vi "Measurement UI.vi"() -> ()   [LabVIEW 2024, in "OneShot-PureTone UI.lvlib"]
uses:
  OneShot-PureTone UI.lvlib
  <vilib>/addons/_XControls/Spectrum with Cursors/Spectrum with Cursors.xctl
  <vilib>/addons/_NISVFA/_Shared subVIs/Data Objects/Data/Data.lvclass
  <vilib>/Addons/_XControls/Waveforms with Cursors/Waveforms with Cursors.xctl
  <vilib>/addons/_NISVFA/_Shared subVIs/Controls/svc_Window.ctl
  <vilib>/addons/_NISVFA/_Shared subVIs/Data Objects/Data/Data.lvclass/Data.ctl
  <vilib>/addons/_NISVFA/_Shared subVIs/Common/SVL Set dB Reference (1 Ch).vi
  <vilib>/addons/Sound and Vibration/svt_Level/SVL AC & DC Level (Time) (1 Ch).vi
  <vilib>/addons/Sound and Vibration/svt_Single Tone Measurements/SVT Spurious Free Dynamic Range (Frequency) (1 Ch).vi
  <vilib>/addons/_NISVFA/_Shared subVIs/Data Objects/Y (Complex) (DBL)/SV Convert Complex Spectrum to Data Object.vi
  <vilib>/addons/_NISVFA/_Shared subVIs/Common/SVL Set dB Reference (variant).vi
  <vilib>/addons/_NISVFA/_Shared subVIs/Common/svc_Get SV Channel Info.vi
  <vilib>/Analysis/baseanly.llb/Mean.vi
  <vilib>/Analysis/baseanly.llb/Mean (DBL).vi
  <vilib>/addons/_NISVFA/_Shared subVIs/Windowing/svfa_Scaled Time Domain Window (Array).vi
  <vilib>/addons/_NISVFA/_Spectrum Processing/SVFA Get Spectrum Subset.vi
  <vilib>/addons/_NISVFA/_Spectrum Processing/SVFA Get Spectrum Subset (Complex) (1 Ch).vi
  <vilib>/addons/_NISVFA/_Shared subVIs/Common/svc_Window Parameters.vi
  <vilib>/addons/_NISVFA/_Shared subVIs/Common/svc_Extract Single Tone Information (complex).vi
  <vilib>/addons/_NISVFA/_Shared subVIs/Common/svc_Check Frequency Range in Spectrum.vi
  <vilib>/addons/_NISVFA/_Spectrum Processing/SVFA Unit Conversion.vi
  <vilib>/addons/_NISVFA/_Spectrum Processing/SVFA Unit Conversion (Complex) (1 Ch).vi
  <vilib>/addons/_NISVFA/_Spectrum Processing/SVFA Spectrum Peak Search.vi
  <vilib>/addons/_NISVFA/_Spectrum Processing/SVFA Spectrum Peak Search (1 Ch).vi
  <vilib>/addons/_NISVFA/_Shared subVIs/Common/svc_Spectrum Units.vi
  <vilib>/addons/_NISVFA/_Shared subVIs/Common/sv_Get NI Property Name String.vi
  <vilib>/addons/_NISVFA/_Shared subVIs/Data Objects/Data/Write Data Attributes.vi
  <vilib>/addons/_NISVFA/_Shared subVIs/Common/svc_Unit Label to Engineering Units.vi
  <vilib>/addons/_NISVFA/_Shared subVIs/Common/svc_Engineering Units to Unit Label.vi
  <vilib>/addons/_NISVFA/_Spectrum Processing/subVIs/svfa_Spectrum Info Window to windowTd Type Def.vi
  <vilib>/Analysis/4window.llb/Force Window.vi
  <vilib>/Analysis/4window.llb/Force Window (DBL).vi
  <vilib>/Analysis/4window.llb/Exponential Window.vi
  <vilib>/Analysis/4window.llb/Exponential Window (DBL).vi
  <vilib>/addons/_NISVFA/_Shared subVIs/Common/svc_Build Unit Label for Frequency Range.vi
  <vilib>/addons/_NISVFA/_Spectrum Processing/SVFA Get Tone Amplitude and Phase (1 Ch).vi
  <vilib>/addons/_NISVFA/_Spectrum Processing/subVIs/svfa_Compute Complex Spectrum for Export.vi
  <vilib>/addons/_NISVFA/_Shared subVIs/Common/svc_Check Frequency Range in Bandwidth.vi
  <vilib>/addons/_NISVFA/_Shared subVIs/Common/svc_Convert Start and Stop to Start Index and Length.vi
  <vilib>/addons/_NISVFA/_Shared subVIs/Common/svc_Log View for Spectrum (1Ch).vi
  <vilib>/addons/_NISVFA/_Spectrum Processing/SVFA Unit Conversion (1 Ch).vi
  <vilib>/addons/_NISVFA/_Shared subVIs/Common/svc_Complex Datatype Defaults.vi
  <vilib>/addons/_NISVFA/_Spectrum Processing/subVIs/svfa_Spectrum Peak Search.vi
  <vilib>/addons/_NISVFA/_Shared subVIs/Common/svc_Format Value (DBL).vi
  <vilib>/addons/_NISVFA/_Shared subVIs/Common/svc_Get Weighting Enum and Labels.vi
  <vilib>/addons/_NISVFA/_Shared subVIs/Common/svc_Surround NonAlpha String with Parentheses.vi
  <vilib>/dlg_ctls.llb/Space Constant.vi
  <vilib>/addons/_NISVFA/_Shared subVIs/Data Objects/Data/Read Data Attributes.vi
  <vilib>/addons/_NISVFA/_Spectrum Processing/subVIs/svfa_Window Frequency Response.vi
  <vilib>/addons/_NISVFA/_Spectrum Processing/subVIs/svfa_Window Frequency Response (double array).vi
  <vilib>/Analysis/baseanly.llb/Dot Product.vi
  <vilib>/Analysis/baseanly.llb/Complex Dot Product.vi
  <vilib>/addons/_NISVFA/_Shared subVIs/Common/svc_Unwrap Phase.vi
  <vilib>/addons/_NISVFA/_Shared subVIs/Common/svc_Convert Spectrum Array to dB.vi
  <vilib>/addons/_NISVFA/_Spectrum Processing/subVIs/svfa_Conversion Utility (spectrum info).vi
  <vilib>/addons/_NISVFA/_Spectrum Processing/subVIs/svfa_Peak Rough Search Indices.vi
  <vilib>/addons/_NISVFA/_Shared subVIs/Common/svc_Unit Label Lexical Class.vi
  <vilib>/addons/_NISVFA/_Spectrum Processing/subVIs/svfa_Rect Window Frequency Response.vi
  <vilib>/addons/_NISVFA/_Spectrum Processing/subVIs/svfa_Cosine Window Coefficients.vi
  <vilib>/addons/_NISVFA/_Spectrum Processing/subVIs/svfa_Peak to RMS to Peak2Peak.vi
  <vilib>/addons/_NISVFA/_Spectrum Processing/subVIs/svfa_Mag to Mag2.vi
  <vilib>/addons/_NISVFA/_Spectrum Processing/subVIs/svfa_Linear to dB.vi
  <vilib>/addons/_NISVFA/_Spectrum Processing/subVIs/svfa_dBrefA to dBrefB.vi
  <vilib>/addons/_NISVFA/_Spectrum Processing/subVIs/svfa_Spectrum to Spectral Density.vi
  <vilib>/addons/_NISVFA/_Shared subVIs/Data Objects/Y (Complex) (DBL)/Y (Complex) (1 Ch).lvclass
  <vilib>/addons/_NISVFA/_Shared subVIs/Common/svc_Caller VI Returned in Error Source.vi
  <vilib>/addons/_NISVFA/_Shared subVIs/Common/svc_Get Window Info.vi
  <vilib>/Analysis/0measdsp.llb/Scaled Time Domain Window.vi
  <vilib>/Analysis/0measdsp.llb/Scaled Time Domain Window (DBL).vi
  <vilib>/Utility/error.llb/Error Cluster From Error Code.vi
  <vilib>/Analysis/baseanly.llb/Std Deviation and Variance.vi
  <vilib>/addons/Sound and Vibration/svt_Single Tone Measurements/SVT Gain (Time) (1 Ch).vi
  <vilib>/addons/Sound and Vibration/svt_Distortion/SVT THD and Harmonic Components (Frequency) (1 Ch).vi
  <vilib>/addons/Sound and Vibration/svt_Distortion/SVT SNR without Harmonics (Frequency) (1 Ch).vi
  <vilib>/addons/Sound and Vibration/svt_Single Tone Measurements/SVT Dynamic Range (Frequency) (1 Ch).vi
  <vilib>/addons/Sound and Vibration/svt_Distortion/subVIs/sv_Check Data Valid (Audio) (1 Ch).vi
  <vilib>/addons/_NISVFA/_Shared subVIs/Common/svc_Convert Frequency to Frequency String.vi
  <vilib>/Analysis/4window.llb/window parameters.vi
  <vilib>/Analysis/4window.llb/Window Properties.vi
  <vilib>/Analysis/4window.llb/Window Properties by Name.vi
  <vilib>/addons/_NISVFA/_Spectrum Processing/subVIs/svfa_Spectrum Peak Tone Search and Estimation (complex).vi
  <vilib>/measure/masignal.llb/Tones and Noise Waveform.vi
  <vilib>/addons/_NISVFA/_Shared subVIs/Common/svc_FFT with Window.vi
  <vilib>/Analysis/1siggen.llb/Square Wave.vi
  <vilib>/addons/_NISVFA/_Spectrum Processing/subVIs/svfa_Three Finger Peak Search.vi
  <vilib>/addons/Sound and Vibration/svt_Distortion/subVIs/sv_Peak View Amplitude (1 Ch).vi
  <vilib>/addons/_NISVFA/_Shared subVIs/Data Objects/Y (Complex) (DBL)/Write Y.vi
  <vilib>/addons/_NISVFA/_Shared subVIs/Spectrum Info/sv_Convert Spectrum Info to Variant Attributes.vi
  <vilib>/addons/Sound and Vibration/svt_Distortion/SoundVib_Distortion.lvlib
  <vilib>/addons/Sound and Vibration/svt_Single Tone Measurements/SoundVib_SingleTone.lvlib
panel:
  out "Waveforms with Cursors":waveform(dbl)[](xcontrol)
  out "THD maximum harmonic out":i32=9 min=-1 max=1000
  out "measurement subset dt":dbl
  out "measurement subset t0":dbl
  out "acquired response dt":dbl
  out "acquired response t0":dbl
  out "measurement subset":dbl[](array[numeric])
  out "acquired response":dbl[](array[numeric])
  out "band stop (Hz) out":dbl=20000.0 format="%.2f"
  out "band start (Hz) out":dbl=20.0 format="%.2f"
  out "detected frequency (Hz)":dbl=1000.0 min=20.0 max=100000.0 step=1.0 format="%.2f"
  out "Spectrum with Cursors":refnum<class "Data.lvclass">(xcontrol)
  out "detected amplitude":dbl=1.0 format="%.3g"
  in  "Tab Control":T1(tab)
  in  "output channel":string="Dev1/ao0"
  in  "ao pure tone channel (I/O)":tag caption="output channel"
  in  "AI range":dbl=-3.0 caption="ai range" format="±  %.3g V"
  in  "ai response channel (I/O)":tag caption="input channel"
  in  "input channel":string="Dev1/ai0"
  in  "sample rate (Hz)":dbl=51200.0 caption="sample rate" min=0.0 format="%#.2p Hz"
  in  "settle cycles":dbl=2.0 min=0.0 format="%#_g cycles"
  in  "settle time (s)":dbl=0.01 caption="settling" format="%#_3g s"
  in  "measurement cycles":dbl=20.0 min=1.0 format="%#_g cycles"
  in  "measurement duration (s)":dbl=0.1 caption="measurement" format="%#_3g s"
  in  "frequency (Hz)":dbl=997.0 caption="frequency" format="%_4f Hz"
  in  "amplitude":dbl=1.0 format="%_4g V"
  in  "THD maximum harmonic":i32=9 caption="THD max harmonic" min=-1 max=1000
  in  "band start (Hz)":dbl=20.0 caption="band start" format="%#_3p Hz"
  in  "band stop (Hz)":dbl=20000.0 caption="band stop" format="%#_3p Hz"
  in  "full scale (V pk)":dbl=2.0 caption="full scale" format="%#_3g V"
  out "SFDR (dB)":dbl caption="SFDR" format="%.1f dB"
  out "Dynamic Range (dB FS)":dbl caption="dynamic range" format="%.1f dB FS"
  out "THD+N (dB)":dbl caption="THD+N" format="%.1f dB"
  out "THD (%)":dbl caption="THD" format="%_4f %"
  out "SNR (dB)":dbl caption="SNR" format="%.1f dB"
  out "fundamental frequency (Hz)":dbl caption="fundamental frequency" format="%_6g Hz"
  out "fundamental amplitude (V)":dbl caption="fundamental amplitude" format="%_6g V"
  out "gain (dB)":dbl caption="gain" format="%.3f dB"
  out "THD (dB)":dbl caption="THD" format="%.1f dB"
  out "processing error":errorcluster
  # "These settings can be changed to remeasure \ndistortion and noise on existing response data."
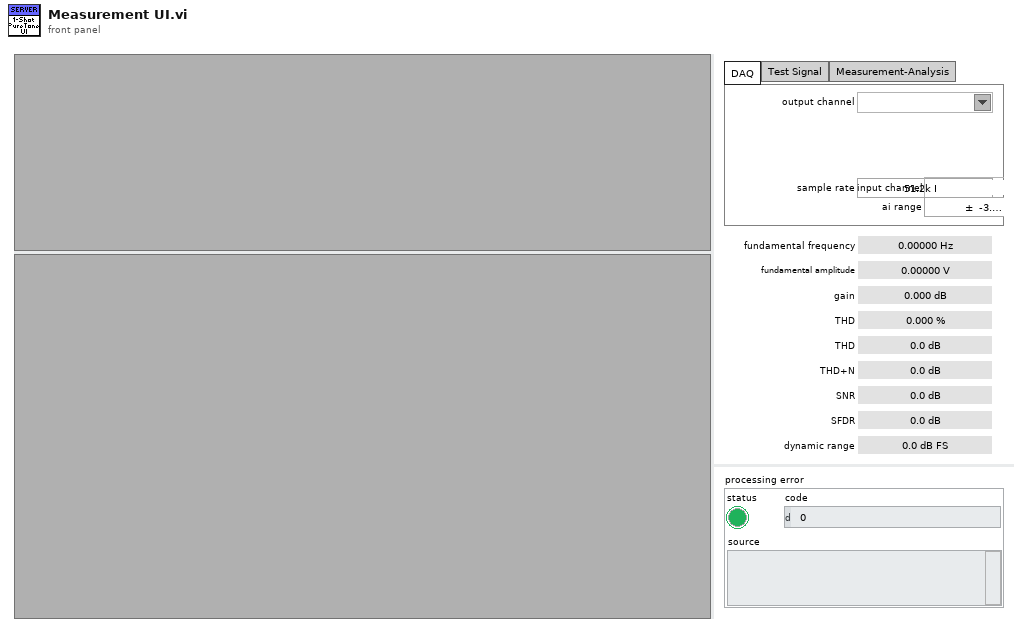
[diagram p1: front panel]
types:
  T1 = enum32{"DAQ", "Test Signal", "Measurement-Analysis"}
  T2 = cluster{"SNR units":enum16{"dB", "linear ratio", "%"}, "detected fundamental amplitude units":enum16{"EU rms", "EU peak", "EU peak-peak"}}
  T3 = cluster{"THD units":enum16{"dB", "linear ratio", "%"}, "harmonic component amplitude units":enum16{"EU rms", "EU peak", "EU peak-peak", "dB ref fund"}, "detected fundamental amplitude units":enum16{"EU rms", "EU peak", "EU peak-peak"}}
  T4 = cluster{"gain units":enum16{"dB", "linear ratio"}, "detected fundamental amplitude units":enum16{"EU rms", "EU peak", "EU peak-peak"}}
  T5 = typedef "svc_Window.ctl" = u32
  T6 = cluster{"band start (Hz)":dbl, "band stop (Hz)":dbl}
  T7 = typedef "svc_Spectrum Info.ctl" = cluster{"channel name":string, "description":string, "x-axis units":T8, "spectral info":cluster{"spectrum type":T9, "linear/dB":enum16{"linear", "dB"}, "window":u16, "window size":i32, "FFT size":i32}, "engineering units":T10, "custom label":string, "dB reference [EU]":dbl, "peak units":enum16{"rms", "peak", "peak-peak"}, "weighting filter":T11, "spectral density?":bool, "unit label":string, "spectrum skewed?":bool, "complimentary spectrum units":T12}
  T8 = typedef "svc_X-Axis Units.ctl" = u16
  T9 = typedef "svc_Spectrum Type.ctl" = enum16{"FFT Spectrum [complex]", "Amplitude [Magnitude]", "Power [Magnitude^2]", "Cross Spectrum [complex]", "Frequency Response [Complex]"}
  T10 = typedef "svc_Engineering Units Text Ring.ctl" = u16
  T11 = typedef "svc_Weighting Filter Text Ring.ctl" = u16
  T12 = typedef "svc_Complimentary Spectrum Units.ctl" = enum16{"none", "radians", "degrees", "cycles", "imaginary"}
  T13 = cluster{"complex spectrum response":cluster{"f0":dbl, "df":dbl, "complex spectrum":cdb[]}, "spectrum info":T7}
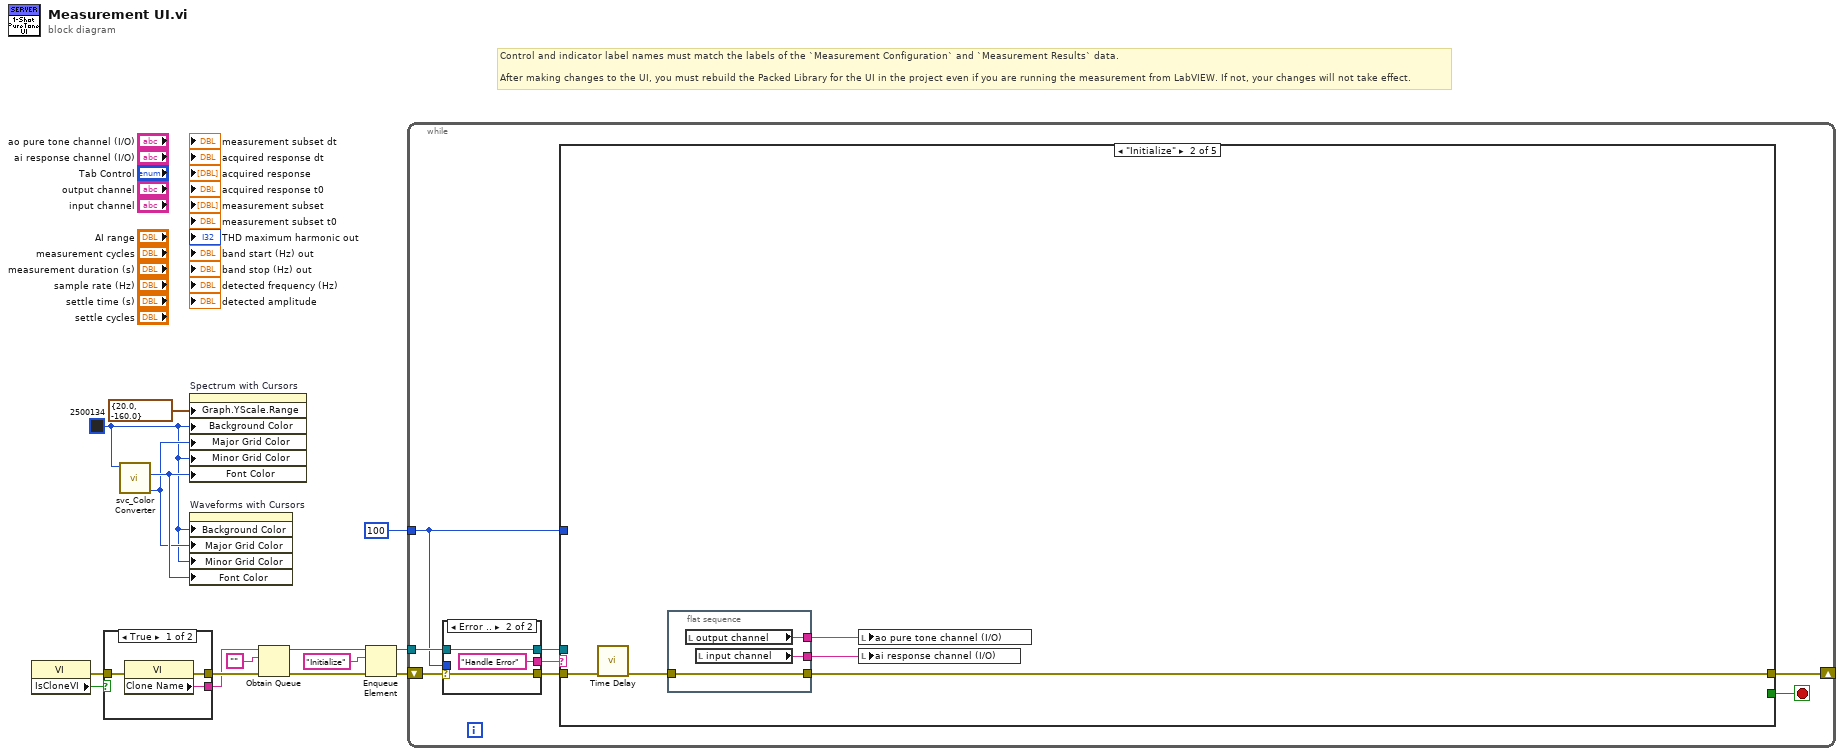
[diagram p0: block diagram]
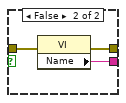
[diagram p2: hidden frame]
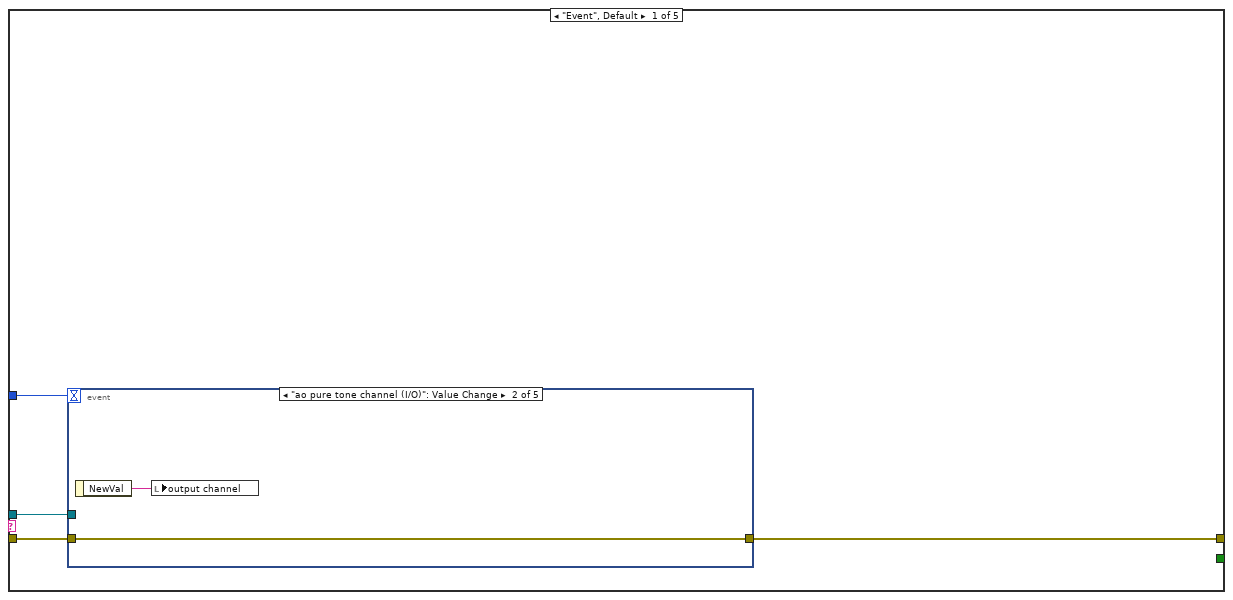
[diagram p3: hidden frame]
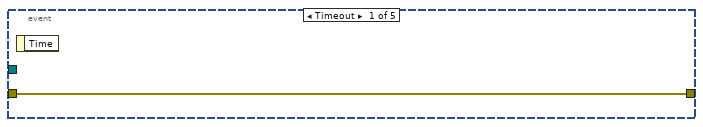
[diagram p4: hidden frame]
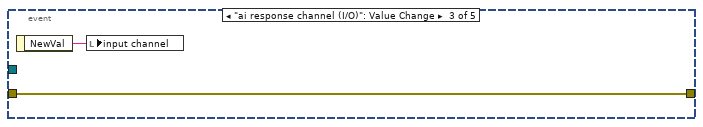
[diagram p5: hidden frame]
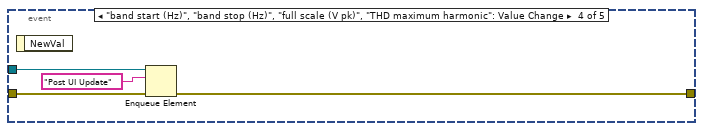
[diagram p6: hidden frame]
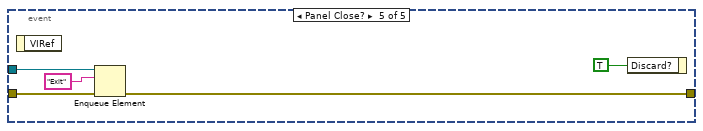
[diagram p7: hidden frame]
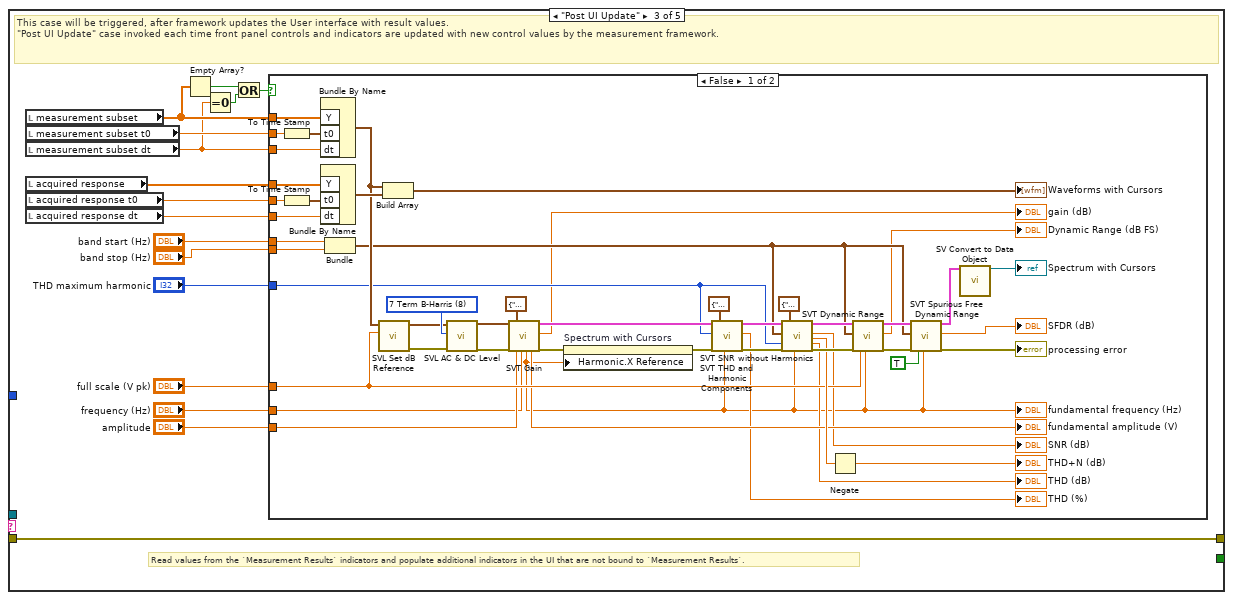
[diagram p8: hidden frame]
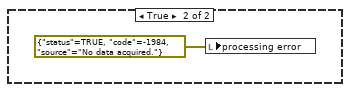
[diagram p9: hidden frame]
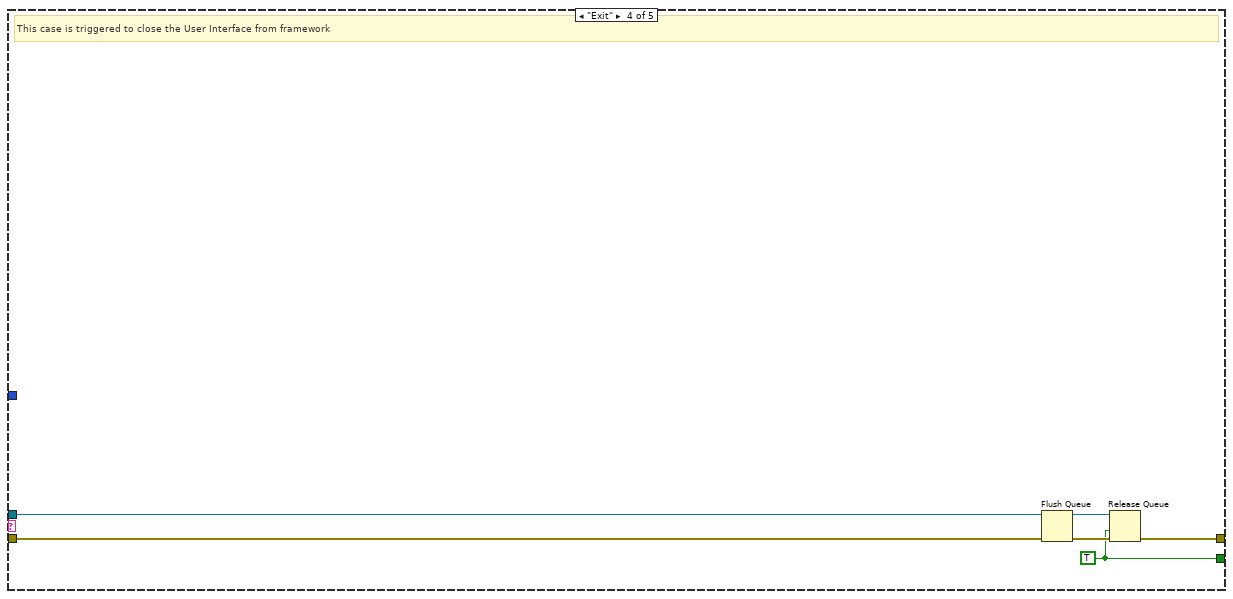
[diagram p10: hidden frame]
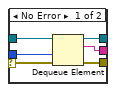
[diagram p12: hidden frame]
diagram:
  w3 = u32 2500134 ("Colors:Background")
  # "Control and indicator label names must match the labels of the `Measurement Configuration` and `Measurement Results` data. \n\nAfter making changes to the UI, you must rebuild the Packed Library for the UI in the project even if you are running the measurement from LabVIEW. If not, your changes will not take effect."
  n1 = property class="VI"() -> (error out=w6:errorcluster, "IsCloneVI"=w7:bool)  [unwired: 2 in, 1 out]
  n2 = case shown="True" w7 {
    tunnel: [w18 w21] -> w15
    tunnel: [w17 w20] -> w14
    tunnel: w6 -> [w16 w19]
    frame True {
      n3 = property class="VI"(error in=w16) -> (error out=w18:errorcluster, "Clone Name"=w17:string)  [unwired: 1 in, 1 out]
    }
    frame False {
      n4 = property class="VI"(error in=w19) -> (error out=w21:errorcluster, "Name"=w20:string)  [unwired: 1 in, 1 out]
    }
  }
  n5 = call <vilib>:"svc_Color Converter.vi"("BG color"=w3) -> ("low contrast"=w4:u32, "maximum contrast"=w5:u32)  [unwired: 7 in, 2 out]
  n6 = property on="Spectrum with Cursors" class="Spectrum with Cursors (strict)"("Graph.YScale.Range"=cluster{"max":dbl, "min":dbl} {"max"=20.0, "min"=-160.0} ("YScale:Range"), "Background Color"=w3, "Major Grid Color"=w4, "Minor Grid Color"=w3, "Font Color"=w5) -> ()  [unwired: 2 in, 2 out]
  n7 = property on="Waveforms with Cursors" class="Waveforms with Cursors (strict)"("Background Color"=w3, "Major Grid Color"=w4, "Minor Grid Color"=w3, "Font Color"=w5) -> ()  [unwired: 2 in, 2 out]
  n8 = Obtain Queue(name (unnamed)=w14, element data type="", error in (no error)=w15) -> (queue out=w11:refnum<queue>, error out=w13:errorcluster)  [unwired: 2 in, 1 out]
  n9 = Enqueue Element(queue=w11, element="Initialize", error in (no error)=w13) -> (queue out=w10:refnum<queue>, error out=w12:errorcluster)  [unwired: 1 in, 1 out]
  n10 = while {
    shift-right: [w24] -> _
    shift-left: w12 -> [w29]
    tunnel: w10 -> [w27]
    tunnel: 100 -> [w22]
    stop <- w23 stop-if-true
    n11 = case shown="Error .." w29 {
      selector: w29 -> [w134 w137]
      tunnel: [w133 w137] -> w28
      tunnel: w27 -> [w132 w136]
      tunnel: [w131 w136] -> w26
      tunnel: [w130 "Handle Error"] -> w25
      tunnel: w22 -> [w129 _]
      frame No Error {
        n12 = Dequeue Element(queue=w132, timeout in ms (-1)=w129, error in (no error)=w134) -> (queue out=w131:refnum<queue>, element=w130:string, error out=w133:errorcluster)  [unwired: 1 out]
      }
      frame Error {
      }
    }
    n13 = case shown="\"Initialize\"" w25 {
      tunnel: w28 -> [w32 w52 w71 w127 w128]
      tunnel: w26 -> [w31 _ _ w126 _]
      tunnel: [w33 w51 w71 w123 w128] -> w24
      tunnel: [_ _ _ w122 _] -> w23
      tunnel: w22 -> [w30 _ _ _ _]
      frame "Event", Default {
        n14 = event shown="[1] \"ao pure tone channel (I/O)\": Value Change" {
          selector: _ -> [_ _ _ _ _]
          dyn-events: _ -> [_ _ _ _ _]
          timeout: w30 -> [_ _ _ _ _]
          tunnel: [w34 w35 w37 w41 w45] -> w33
          tunnel: w32 -> [w34 w35 w37 w42 w46]
          tunnel: w31 -> [_ _ _ w40 w44]
          event Timeout {
            n15 = event-data() -> ()  [unwired: 1 in, 1 out]
          }
          event "ao pure tone channel (I/O)": Value Change {
            n16 = event-data() -> ("NewVal"=w36:tag)  [unwired: 1 in]
            n17 = local write "output channel"(w36) -> ()
          }
          event "ai response channel (I/O)": Value Change {
            n18 = event-data() -> ("NewVal"=w38:tag)  [unwired: 1 in]
            n19 = local write "input channel"(w38) -> ()
          }
          event "band start (Hz)", "band stop (Hz)", "full scale (V pk)", "THD maximum harmonic": Value Change {
            n20 = event-data() -> ()  [unwired: 1 in, 1 out]
            n21 = Enqueue Element(queue=w40, element="Post UI Update", error in (no error)=w42) -> (error out=w41:errorcluster)  [unwired: 1 in, 2 out]
          }
          event Panel Close? {
            n22 = event-data() -> ()  [unwired: 1 in, 1 out]
            n23 = Enqueue Element(queue=w44, element="Exit", error in (no error)=w46) -> (error out=w45:errorcluster)  [unwired: 1 in, 2 out]
            n24 = event-data("Discard?"=TRUE) -> ()  [unwired: 1 in, 1 out]
          }
        }
      }
      frame "Initialize" {
        n25 = call "Time Delay"("error in (no error)"=w52) -> ("error out"=w50:errorcluster)  [unwired: 10 in]
        n26 = flat-sequence {
          tunnel: w50 -> [w55]
          tunnel: [w55] -> w51
          tunnel: [w54] -> w49
          tunnel: [w53] -> w48
          frame #0 {
            n27 = local read "output channel"() -> (w54:string)
            n28 = local read "input channel"() -> (w53:string)
          }
        }
        n29 = local write "ao pure tone channel (I/O)"(w49) -> ()
        n30 = local write "ai response channel (I/O)"(w48) -> ()
      }
      frame "Post UI Update" {
        # "Read values from the `Measurement Results` indicators and populate additional indicators in the UI that are not bound to `Measurement Results`."
        # "This case will be triggered, after framework updates the User interface with result values.\n\"Post UI Update\" case invoked each time front panel controls and indicators are updated with new control values by the measurement framework."
        n31 = local read "measurement subset"() -> (w60:dbl[])
        n32 = local read "measurement subset t0"() -> (w67:dbl)
        n33 = local read "measurement subset dt"() -> (w58:dbl)
        n34 = local read "acquired response"() -> (w70:dbl[])
        n35 = local read "acquired response t0"() -> (w68:dbl)
        n36 = local read "acquired response dt"() -> (w69:dbl)
        n37 = Empty Array?(array=w60) -> (empty?=w59:bool)
        n38 = Equal To 0?(x=w58) -> (x = 0?=w56:bool)
        n39 = Or(x=w59, y=w56) -> (x .or. y?=w57:bool)
        n40 = case shown="False" w57 {
          tunnel: w70 -> [w120 _]
          tunnel: w69 -> [w119 _]
          tunnel: w58 -> [w118 _]
          tunnel: w68 -> [w115 _]
          tunnel: w67 -> [w114 _]
          tunnel: "band start (Hz)" -> [w92 _]
          tunnel: "band stop (Hz)" -> [w91 _]
          tunnel: "THD maximum harmonic" -> [w89 _]
          tunnel: "full scale (V pk)" -> [w88 _]
          tunnel: "amplitude" -> [w87 _]
          tunnel: "frequency (Hz)" -> [w86 _]
          tunnel: w60 -> [w75 _]
          frame False {
            w112 = T5 8 items=["None"=0, "Hanning"=1, "Hamming"=2, "Blackman-Harris"=3, "Exact Blackman"=4, "Blackman"=5, "Flat Top"=6, "4 Term B-Harris "=7, "7 Term B-Harris"=8, "Low Sidelobe"=9, "Force"=64, "Exponential"=65, "Blackman Nuttall"=11, "Triangle"=30, "Bartlett-Hanning"=31, "Bohman"=32, "Parzen"=33, "Welch"=34, "Kaiser"=60, "Dolph-Chebyshev"=61, "Gaussian"=62] ("window")
            n41 = To Time Stamp(1:w114) -> (0:w117:timestamp)
            n42 = To Time Stamp(1:w115) -> (0:w116:timestamp)
            n43 = Bundle By Name("Y"=w75, "t0"=w117, "dt"=w118) -> (w93:waveform(dbl))  [unwired: 1 in]
            n44 = Bundle By Name("Y"=w120, "t0"=w116, "dt"=w119) -> (w113:waveform(dbl))  [unwired: 1 in]
            n45 = Bundle("band start (Hz)"=w92, "band stop (Hz)"=w91) -> (w90:T6)  [unwired: 1 in]
            n46 = call-poly <vilib>:"SVL Set dB Reference.vi"("dB reference [EU]"=w88, "scaled signal in [EU]"=w93) -> ("error out"=w110:errorcluster, "scaled signal out [EU]"=w108:waveform(dbl))  [unwired: 8 in]
            n47 = Build Array(w93, w113) -> (→"Waveforms with Cursors":waveform(dbl)[])
            n48 = call-poly <vilib>:"SVL AC & DC Level.vi"("scaled signal [EU]"=w108, "window"=w112, "error in (no error)"=w110) -> ("AC signal [EU]"=w109:waveform(dbl), "error out"=w111:errorcluster)  [unwired: 11 in, 4 out]
            n49 = call-poly <vilib>:"SVT Gain.vi"("scaled signal [EU]"=w109, "error in (no error)"=w111, "desired units"=T4 {"gain units"=enum."dB", "detected fundamental amplitude units"=enum."EU peak"}, "amplitude [EU peak]"=w87, "expected fundamental frequency [Hz]"=w86) -> ("detected fundamental\nfrequency [Hz]"=w72:dbl, "detected fundamental\namplitude"=→"fundamental amplitude (V)":dbl, "complex spectrum"=w95:T13, "gain"=→"gain (dB)":dbl, "error out"=w74:errorcluster)  [unwired: 9 in, 1 out]
            "fundamental frequency (Hz)" <- w72
            n50 = property on="Spectrum with Cursors" class="Spectrum with Cursors (strict)"(error in=w74, "Harmonic.X Reference"=w72) -> (error out=w73:errorcluster)  [unwired: 1 in, 1 out]
            n51 = call-poly <vilib>:"SVT THD and Harmonic Components.vi"("complex spectrum"=w95, "maximum harmonic"=w89, "error in (no error)"=w73, "desired units"=T3 {"THD units"=enum."%", "harmonic component amplitude units"=enum."EU peak", "detected fundamental amplitude units"=enum."EU peak"}, "expected fundamental frequency [Hz]"=w72) -> ("complex spectrum"=w100:T13, "THD"=→"THD (%)":dbl, "error out"=w104:errorcluster)  [unwired: 7 in, 5 out]
            n52 = call-poly <vilib>:"SVT SNR without Harmonics.vi"("complex spectrum"=w100, "frequency range"=w90, "maximum harmonic"=w89, "error in (no error)"=w104, "desired units"=T2 {"SNR units"=enum."dB", "detected fundamental amplitude units"=enum."EU rms"}, "expected fundamental frequency [Hz]"=w72) -> ("complex spectrum"=w102:T13, "SNR (without harmonics)"=→"SNR (dB)":dbl, "SINAD"=w101:dbl, "THD"=→"THD (dB)":dbl, "error out"=w105:errorcluster)  [unwired: 6 in, 3 out]
            n53 = Negate(x=w101) -> (-x=→"THD+N (dB)":dbl)
            n54 = call-poly <vilib>:"SVT Dynamic Range.vi"("complex spectrum"=w102, "frequency range"=w90, "error in (no error)"=w105, "full scale amplitude [EU peak]"=w88, "expected fundamental\nfrequency [Hz]"=w72) -> ("dup complex spectrum"=w103:T13, "dynamic range"=→"Dynamic Range (dB FS)":dbl, "error out"=w106:errorcluster)  [unwired: 9 in, 3 out]
            n55 = call-poly <vilib>:"SVT Spurious Free Dynamic Range.vi"("complex spectrum"=w103, "frequency range"=w90, "error in (no error)"=w106, "exclude harmonics"=TRUE, "expected fundamental\nfrequency [Hz]"=w72) -> ("complex spectrum"=w76:T13, "spurious free dynamic range"=→"SFDR (dB)":dbl, "error out"=→"processing error":errorcluster)  [unwired: 7 in, 5 out]
            n56 = call-poly <vilib>:"SV Convert to Data Object.vi"("complex spectrum"=w76) -> ("Spectrum Data"=→"Spectrum with Cursors":refnum<class "Data.lvclass">)  [unwired: 17 in, 1 out]
          }
          frame True {
            n57 = local write "processing error"(errorcluster {"status"=TRUE, "code"=-1984, "source"="No data acquired."} ("processing error")) -> ()
          }
        }
      }
      frame "Exit" {
        w122 = TRUE ("force destroy? (F)")
        # "This case is triggered to close the User Interface from framework"
        n58 = Flush Queue(queue=w126, error in (no error)=w127) -> (queue out=w125:refnum<queue>, error out=w124:errorcluster)  [unwired: 1 out]
        n59 = Release Queue(queue=w125, force destroy? (F)=w122, error in (no error)=w124) -> (error out=w123:errorcluster)  [unwired: 2 out]
      }
      frame "Handle Error" {
      }
    }
  }
